vi "ParseString.vi"(8 "error in (no error)":errorcluster, 10 "Index In":i32, 11 "JSON String":string) -> (0 "error out":errorcluster, 1 "Parsed String":string, 2 "Index Out":i32, 3 "JSON Tree":variant)   [LabVIEW 2013, in "i3-json.lvlib"]
doc: "Use this template to build a VI to use as a subVI."
uses:
  i3-json.lvlib
  JSON Types/JSON Type.ctl
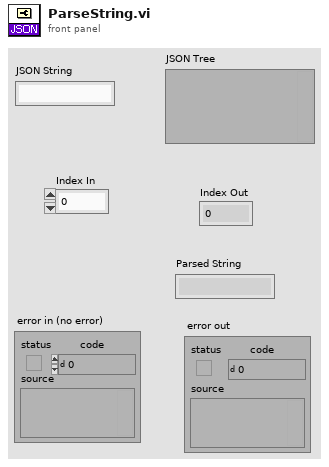
[diagram p1: front panel]
types:
  T1 = typedef "i3-json.lvlib/JSON Type.ctl" = enum8{"JSON Compatible", "JSON Array", "JSON Object", "JSON Null", "Double", "String", "Boolean", "Unknown", "Data JSON string"}
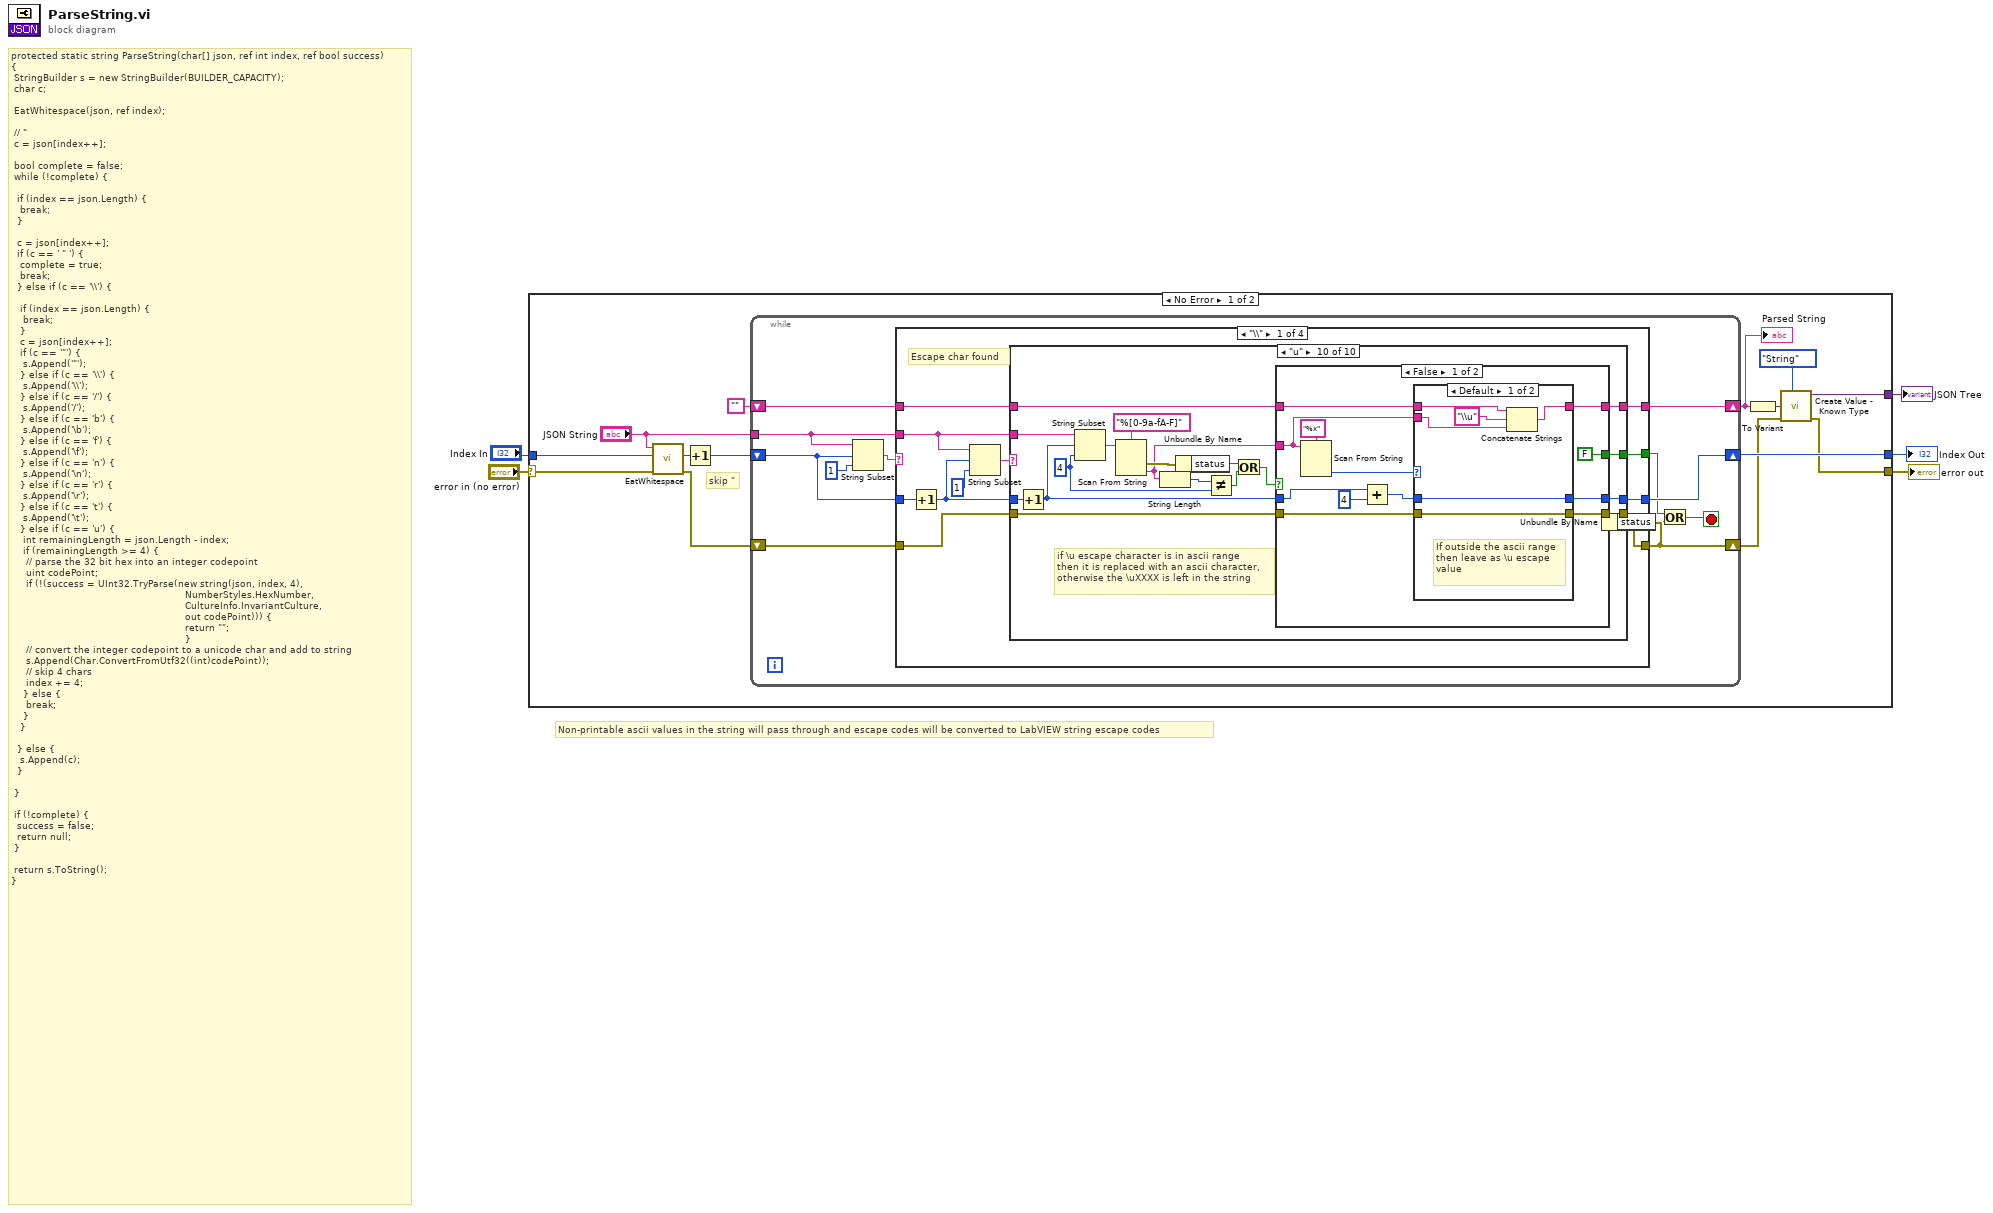
[diagram p0: block diagram]
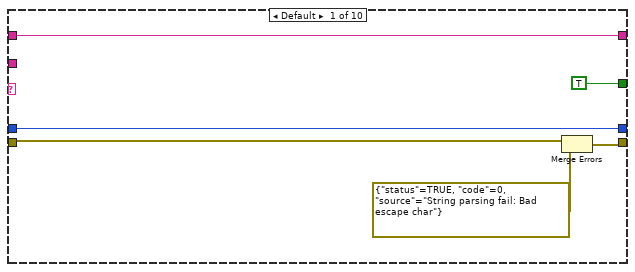
[diagram p2: hidden frame]
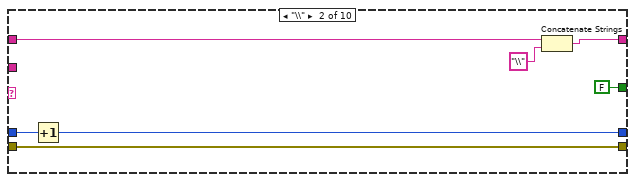
[diagram p3: hidden frame]
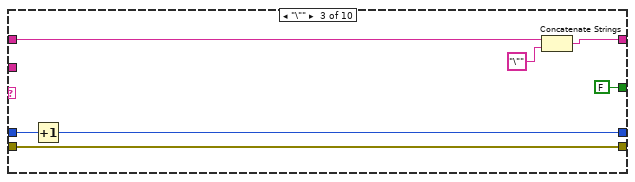
[diagram p4: hidden frame]
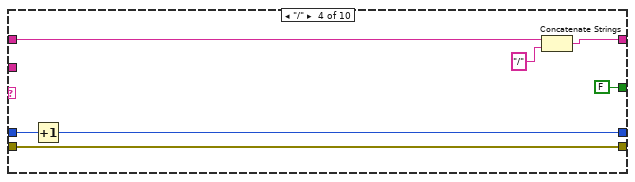
[diagram p5: hidden frame]
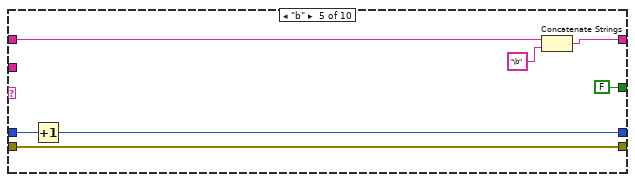
[diagram p6: hidden frame]
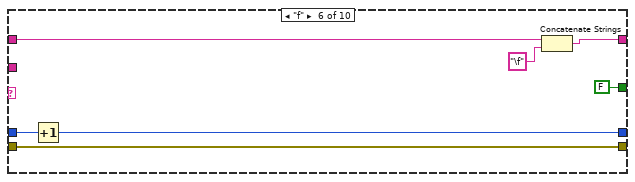
[diagram p7: hidden frame]
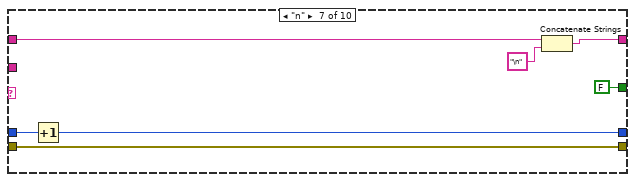
[diagram p8: hidden frame]
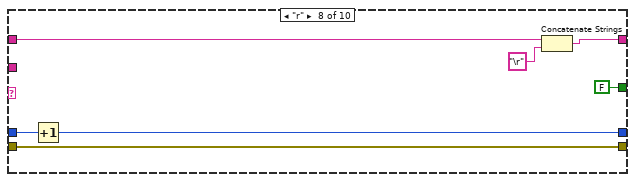
[diagram p9: hidden frame]
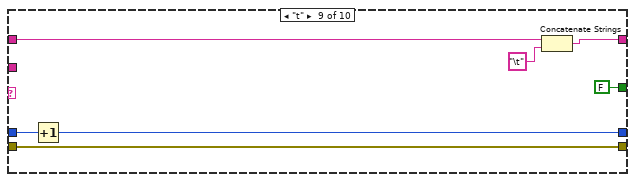
[diagram p10: hidden frame]
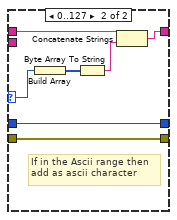
[diagram p11: hidden frame]
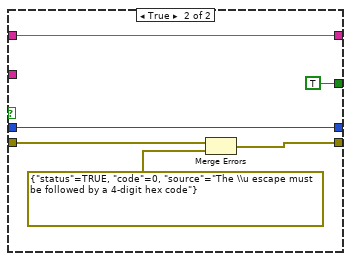
[diagram p12: hidden frame]
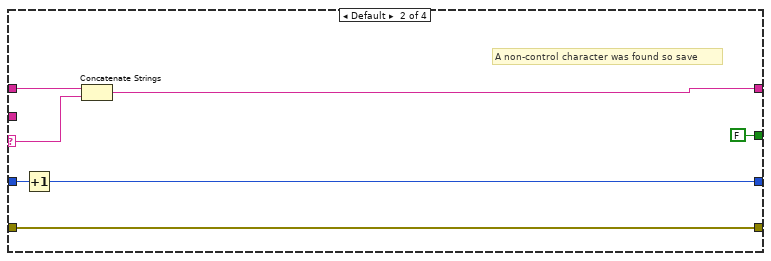
[diagram p13: hidden frame]
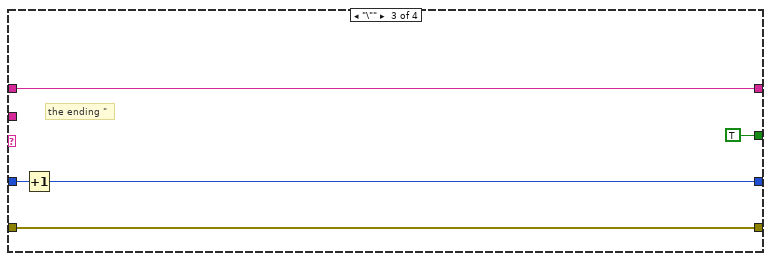
[diagram p14: hidden frame]
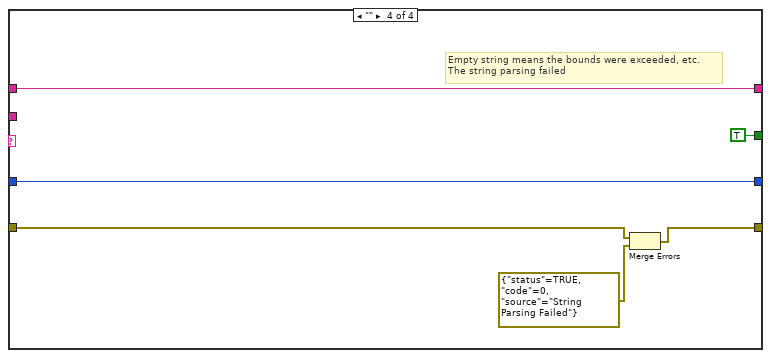
[diagram p15: hidden frame]
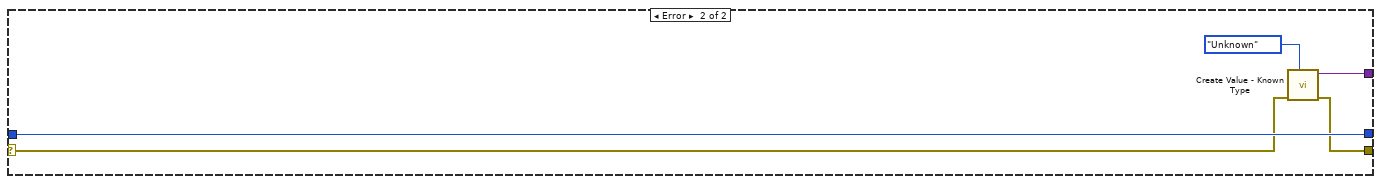
[diagram p16: hidden frame]
diagram:
  # "Non-printable ascii values in the string will pass through and escape codes will be converted to LabVIEW string escape codes"
  # "protected static string ParseString(char[] json, ref int index, ref bool success)\n{\n\tStringBuilder s = new StringBuilder(BUILDER_CAPACITY);\n\tchar c;\n\n\tEatWhitespace(json, ref index);\n\n\t// \"\n\tc = json[index++];\n\n\tbool complete = false;\n\twhile (!complete) {\n\n\t\tif (index == json.Length) {\n\t\t\tbreak;\n\t\t}\n\n\t\tc = json[index++];\n\t\tif (c == ' \" ') {\n\t\t\tcomplete = true;\n\t\t\tbreak;\n\t\t} else if (c == '\\\\') {\n\n\t\t\tif (index == json.Length) {\n\t\t\t\tbreak;\n\t\t\t}\n\t\t\tc = json[index++];\n\t\t\tif (c == '\"') {\n\t\t\t\ts.Append('\"');\n\t\t\t} else if (c == '\\\\') {\n\t\t\t\ts.Append('\\\\');\n\t\t\t} else if (c == '/') {\n\t\t\t\ts.Append('/');\n\t\t\t} else if (c == 'b') {\n\t\t\t\ts.Append('\\b');\n\t\t\t} else if (c == 'f') {\n\t\t\t\ts.Append('\\f');\n\t\t\t} else if (c == 'n') {\n\t\t\t\ts.Append('\\n');\n\t\t\t} else if (c == 'r') {\n\t\t\t\ts.Append('\\r');\n\t\t\t} else if (c == 't') {\n\t\t\t\ts.Append('\\t');\n\t\t\t} else if (c == 'u') {\n\t\t\t\tint remainingLength = json.Length - index;\n\t\t\t\tif (remainingLength >= 4) {\n\t\t\t\t\t// parse the 32 bit hex into an integer codepoint\n\t\t\t\t\tuint codePoint;\n\t\t\t\t\tif (!(success = UInt32.TryParse(new string(json, index, 4),\n                                                          NumberStyles.HexNumber,\n                                                          CultureInfo.InvariantCulture,\n                                                          out codePoint))) {\n\t\t\t\t\t\t                                                    return \"\";\n\t\t\t\t\t                                                     }\n\t\t\t\t\t// convert the integer codepoint to a unicode char and add to string\n\t\t\t\t\ts.Append(Char.ConvertFromUtf32((int)codePoint));\n\t\t\t\t\t// skip 4 chars\n\t\t\t\t\tindex += 4;\n\t\t\t\t} else {\n\t\t\t\t\tbreak;\n\t\t\t\t}\n\t\t\t}\n\n\t\t} else {\n\t\t\ts.Append(c);\n\t\t}\n\n\t}\n\n\tif (!complete) {\n\t\tsuccess = false;\n\t\treturn null;\n\t}\n\n\treturn s.ToString();\n}"
  n1 = case shown="No Error" "error in (no error)" {
    selector: "error in (no error)" -> [w19 w172]
    tunnel: [w10 w173] -> w4
    tunnel: "Index In" -> [w13 w176]
    tunnel: [w12 w176] -> w2
    tunnel: [w8 w174] -> w1
    frame No Error {
      # "skip \""
      n2 = call "EatWhitespace.vi"("error in (no error)"=w19, "Index In"=w13, "JSON String"="JSON String") -> ("error out"=w14:errorcluster, "Index Out"=w18:i32)  [unwired: 6 in, 1 out]
      n3 = Increment(x=w18) -> (x+1=w16:i32)
      n4 = while {
        tunnel: "JSON String" -> [w27]
        shift-right: [w28] -> w6
        shift-left: "" -> [w29]
        shift-right: [w24] -> w12
        shift-left: w16 -> [w25]
        shift-right: [w23] -> w11
        shift-left: w14 -> [w26]
        stop <- w21 stop-if-true
        n5 = String Subset(string=w27, offset (0)=w25, length (rest)=1 ("length (rest)")) -> (substring=w30:string)
        n6 = case shown="\"\\\\\"" w30 {
          selector: w30 -> [_ w159 _ _]
          tunnel: [w33 FALSE TRUE TRUE] -> w22
          tunnel: w29 -> [w39 w160 w164 w171]
          tunnel: [w38 w158 w164 w171] -> w28
          tunnel: w25 -> [w42 w157 w163 w169]
          tunnel: w27 -> [w32 _ _ _]
          tunnel: [w37 w156 w162 w169] -> w24
          tunnel: w26 -> [w35 w154 w161 w168]
          tunnel: [w34 w154 w161 w167] -> w23
          frame "\\" {
            # "Escape char found"
            n7 = Increment(x=w42) -> (x+1=w36:i32)
            n8 = String Subset(string=w32, offset (0)=w36, length (rest)=1 ("length (rest)")) -> (substring=w40:string)
            n9 = case shown="\"u\"" w40 {
              tunnel: w39 -> [w47 w55 w62 w69 w76 w83 w90 w97 w104 w113]
              tunnel: [w47 w54 w61 w68 w75 w82 w89 w96 w103 w109] -> w38
              tunnel: [w46 w51 w58 w65 w72 w79 w86 w93 w100 w107] -> w37
              tunnel: w36 -> [w46 w52 w59 w66 w73 w80 w87 w94 w101 w121]
              tunnel: w35 -> [w44 w50 w57 w64 w71 w78 w85 w92 w99 w112]
              tunnel: [w45 w50 w57 w64 w71 w78 w85 w92 w99 w111] -> w34
              tunnel: [TRUE FALSE FALSE FALSE FALSE FALSE FALSE FALSE FALSE w110] -> w33
              tunnel: w32 -> [_ _ _ _ _ _ _ _ _ w122]
              frame Default {
                n10 = Merge Errors(w44, errorcluster {"status"=TRUE, "code"=0, "source"="String parsing fail: Bad escape char"} ("error out")) -> (w45:errorcluster)
              }
              frame "\\" {
                n11 = Increment(x=w52) -> (x+1=w51:i32)
                n12 = Concatenate Strings(w55, "\\" ("string")) -> (w54:string)
              }
              frame "\"" {
                n13 = Increment(x=w59) -> (x+1=w58:i32)
                n14 = Concatenate Strings(w62, "\"" ("string")) -> (w61:string)
              }
              frame "/" {
                n15 = Increment(x=w66) -> (x+1=w65:i32)
                n16 = Concatenate Strings(w69, "/" ("string")) -> (w68:string)
              }
              frame "b" {
                n17 = Increment(x=w73) -> (x+1=w72:i32)
                n18 = Concatenate Strings(w76, "\b" ("string")) -> (w75:string)
              }
              frame "f" {
                n19 = Increment(x=w80) -> (x+1=w79:i32)
                n20 = Concatenate Strings(w83, "\f" ("string")) -> (w82:string)
              }
              frame "n" {
                n21 = Increment(x=w87) -> (x+1=w86:i32)
                n22 = Concatenate Strings(w90, "\n" ("string")) -> (w89:string)
              }
              frame "r" {
                n23 = Increment(x=w94) -> (x+1=w93:i32)
                n24 = Concatenate Strings(w97, "\r" ("string")) -> (w96:string)
              }
              frame "t" {
                n25 = Increment(x=w101) -> (x+1=w100:i32)
                n26 = Concatenate Strings(w104, "\t" ("string")) -> (w103:string)
              }
              frame "u" {
                w115 = 4 ("length (rest)")
                # "if \\u escape character is in ascii range\nthen it is replaced with an ascii character,\notherwise the \\uXXXX is left in the string"
                n27 = Increment(x=w121) -> (x+1=w108:i32)
                n28 = String Subset(string=w122, offset (0)=w108, length (rest)=w115) -> (substring=w120:string)
                n29 = Scan From String(format string="%[0-9a-fA-F]", input string=w120) -> (error out=w116:errorcluster, output 1=w106:string)  [unwired: 3 in, 2 out]
                n30 = String Length(string=w106) -> (length=w118:i32)
                n31 = Unbundle By Name(w116) -> ("status"=w105:bool)
                n32 = Not Equal?(x=w118, y=w115) -> (x != y?=w117:bool)
                n33 = Or(x=w105, y=w117) -> (x .or. y?=w114:bool)
                n34 = case shown="False" w114 {
                  tunnel: w113 -> [w131 w149]
                  tunnel: w112 -> [w129 w153]
                  tunnel: [w128 w151] -> w111
                  tunnel: [FALSE TRUE] -> w110
                  tunnel: [w130 w149] -> w109
                  tunnel: w108 -> [w124 w148]
                  tunnel: [w127 w148] -> w107
                  tunnel: w106 -> [w126 _]
                  frame False {
                    n35 = Scan From String(format string="%x", input string=w126) -> (output 1=w132:u32)  [unwired: 3 in, 3 out]
                    n36 = Add(x=w124, y=4) -> (x+y=w123:i32)
                    n37 = case shown="Default" w132 {
                      selector: w132 -> [_ w147]
                      tunnel: w131 -> [w137 w145]
                      tunnel: [w138 w144] -> w130
                      tunnel: w129 -> [w139 w143]
                      tunnel: [w139 w143] -> w128
                      tunnel: [w140 w141] -> w127
                      tunnel: w126 -> [w135 _]
                      tunnel: w123 -> [w140 w141]
                      frame Default {
                        # "If outside the ascii range\nthen leave as \\u escape\nvalue"
                        n38 = Concatenate Strings(w137, "\\u" ("string"), w135) -> (w138:string)
                      }
                      frame 0..127 {
                        # "If in the Ascii range then\nadd as ascii character"
                        n39 = Build Array(w147) -> (w146:u32[])
                        n40 = Byte Array To String(unsigned byte array=w146) -> (string=w142:string)
                        n41 = Concatenate Strings(w145, w142) -> (w144:string)
                      }
                    }
                  }
                  frame True {
                    n42 = Merge Errors(w153, errorcluster {"status"=TRUE, "code"=0, "source"="The \\u escape must be followed by a 4-digit hex code"} ("error in")) -> (w151:errorcluster)
                  }
                }
              }
            }
          }
          frame Default {
            # "A non-control character was found so save"
            n43 = Increment(x=w157) -> (x+1=w156:i32)
            n44 = Concatenate Strings(w160, w159) -> (w158:string)
          }
          frame "\"" {
            # "the ending \""
            n45 = Increment(x=w163) -> (x+1=w162:i32)
          }
          frame "" {
            # "Empty string means the bounds were exceeded, etc.\nThe string parsing failed"
            n46 = Merge Errors(w168, errorcluster {"status"=TRUE, "code"=0, "source"="String Parsing Failed"} ("error out")) -> (w167:errorcluster)
          }
        }
        n47 = Unbundle By Name(w23) -> ("status"=w20:bool)
        n48 = Or(x=w22, y=w20) -> (x .or. y?=w21:bool)
      }
      "Parsed String" <- w6
      n49 = To Variant(anything=w6) -> (Variant=w9:variant)
      n50 = call "Create Value - Known Type.vi"("JSON Type"=JSON_Type."String", "error in (no error)"=w11, "Value"=w9) -> ("error out"=w10:errorcluster, "JSON Tree"=w8:variant)  [unwired: 7 in]
    }
    frame Error {
      n51 = call "Create Value - Known Type.vi"("JSON Type"=JSON_Type."Unknown", "error in (no error)"=w172) -> ("error out"=w173:errorcluster, "JSON Tree"=w174:variant)  [unwired: 8 in]
    }
  }
  "error out" <- w4
  "Index Out" <- w2
  "JSON Tree" <- w1
